vi "sub_DO-all-off-raw-DAQmx.vi"() -> ()   [LabVIEW 2019]
uses:
  _ctrl/rw.ctl
  <vilib>/DAQmx/write.llb/DAQmx Write (Digital 1D Bool NChan 1Samp 1Line).vi
  <vilib>/DAQmx/create/channels.llb/DAQmx Create Channel (DO-Digital Output).vi
  <vilib>/DAQmx/miscellaneous.llb/DAQmx Fill In Error Info.vi
panel:
  out "error out":errorcluster
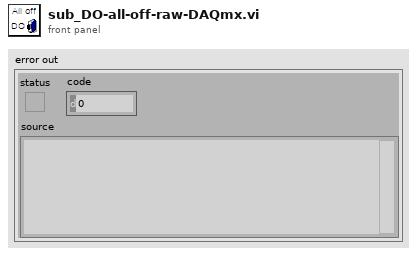
[diagram p1: front panel]
types:
  T1 = typedef "rw.ctl" = enum16{"read", "write"}
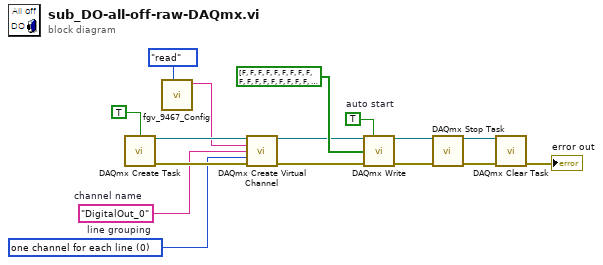
[diagram p0: block diagram]
diagram:
  w5 = 0 items=["one channel for each line", "one channel for all lines"]  # line grouping
  w4 = "DigitalOut_0"  # channel name
  w6 = TRUE  # auto start
  n1 = call <vilib>:"DAQmx Create Task.vi"("auto cleanup"=TRUE) -> ("task out"=w10:refnum<k21>, "error out"=w11:errorcluster)  [unwired: 13 in]
  n2 = call "fgv_9467_Config.vi"("cmd"=rw."read") -> ("cDAQ-9467 Config 2"=w8:tag)  [unwired: 10 in]
  n3 = call-poly <vilib>:"DAQmx Create Virtual Channel.vi"("task in"=w10, "lines"=w8, "name to assign"=w4, "line grouping"=w5, "error in"=w11) -> ("task out"=w3:refnum<k21>, "error out"=w2:errorcluster)  [unwired: 9 in]
  n4 = call-poly <vilib>:"DAQmx Write.vi"("task/channels in"=w3, "auto start"=w6, "data"=bool[] [FALSE, FALSE, FALSE, FALSE, FALSE, FALSE, FALSE, FALSE, FALSE, FALSE, FALSE, FALSE, FALSE, FALSE, FALSE, FALSE, FALSE, FALSE, FALSE, FALSE, FALSE, FALSE, FALSE, FALSE, FALSE, FALSE, FALSE, FALSE, FALSE, FALSE, FALSE, FALSE], "error in"=w2) -> ("task out"=w16:refnum<k21>, "error out"=w15:errorcluster)  [unwired: 9 in, 1 out]
  n5 = call <vilib>:"DAQmx Stop Task.vi"("task/channels in"=w16, "error in"=w15) -> ("task out"=w14:refnum<k21>, "error out"=w13:errorcluster)  [unwired: 12 in]
  n6 = call <vilib>:"DAQmx Clear Task.vi"("task in"=w14, "error in"=w13) -> ("error out"=→"error out":errorcluster)  [unwired: 13 in]
